vi "Read output L.vi"(11 "Y_Limiter in":refnum<class "Y_Limiter.lvclass">) -> (2 "output L":dbl=-100.0 format="%.2f", 3 "Y_Limiter out":refnum<class "Y_Limiter.lvclass">)   [LabVIEW 2019, in "control.lvlib" / "Y_Limiter.lvclass"]
uses:
  Y_Limiter.lvclass
  Y_Limiter.lvclass/Y_Limiter.ctl
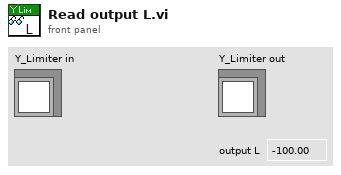
[diagram p1: front panel]
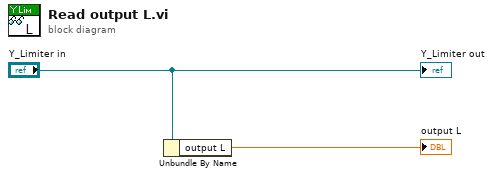
[diagram p0: block diagram]
diagram:
  n1 = Unbundle By Name("Y_Limiter in") -> ("output L"=→"output L":dbl)
  "Y_Limiter out" <- "Y_Limiter in"
